vi "Panel Get Load Info.vi"(2 "file path (dialog if empty)":path) -> (6 "Load Type Out":string(combo), 8 "Nominal Load  Weight Out":string(combo))   [LabVIEW 2012]
uses:
  <vilib>/Utility/miscctls.llb/LVComboBoxStrsAndValuesArrayTypeDef.ctl
  <vilib>/Utility/file.llb/Read From Spreadsheet File (string).vi
panel:
  in  "error IO":errorcluster
  in  "Nominal Load  Weight (Select or Enter Value)":string(combo)
  in  "Load Type (Select or Enter Value)":string(combo)
  in  "stop":bool
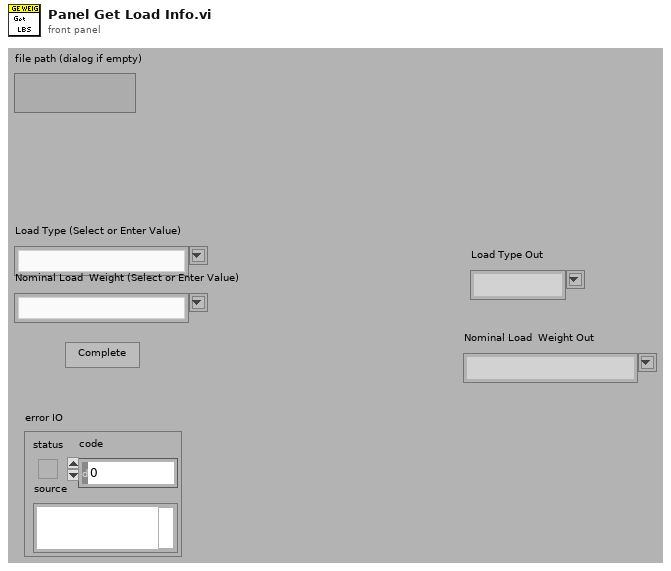
[diagram p1: front panel]
types:
  T1 = typedef "LVComboBoxStrsAndValuesArrayTypeDef.ctl" = cluster{"String":string, "Value":string}[]
  T2 = enum32{"Invalid", "Standard", "Closed", "Hidden", "Minimized", "Maximized"}
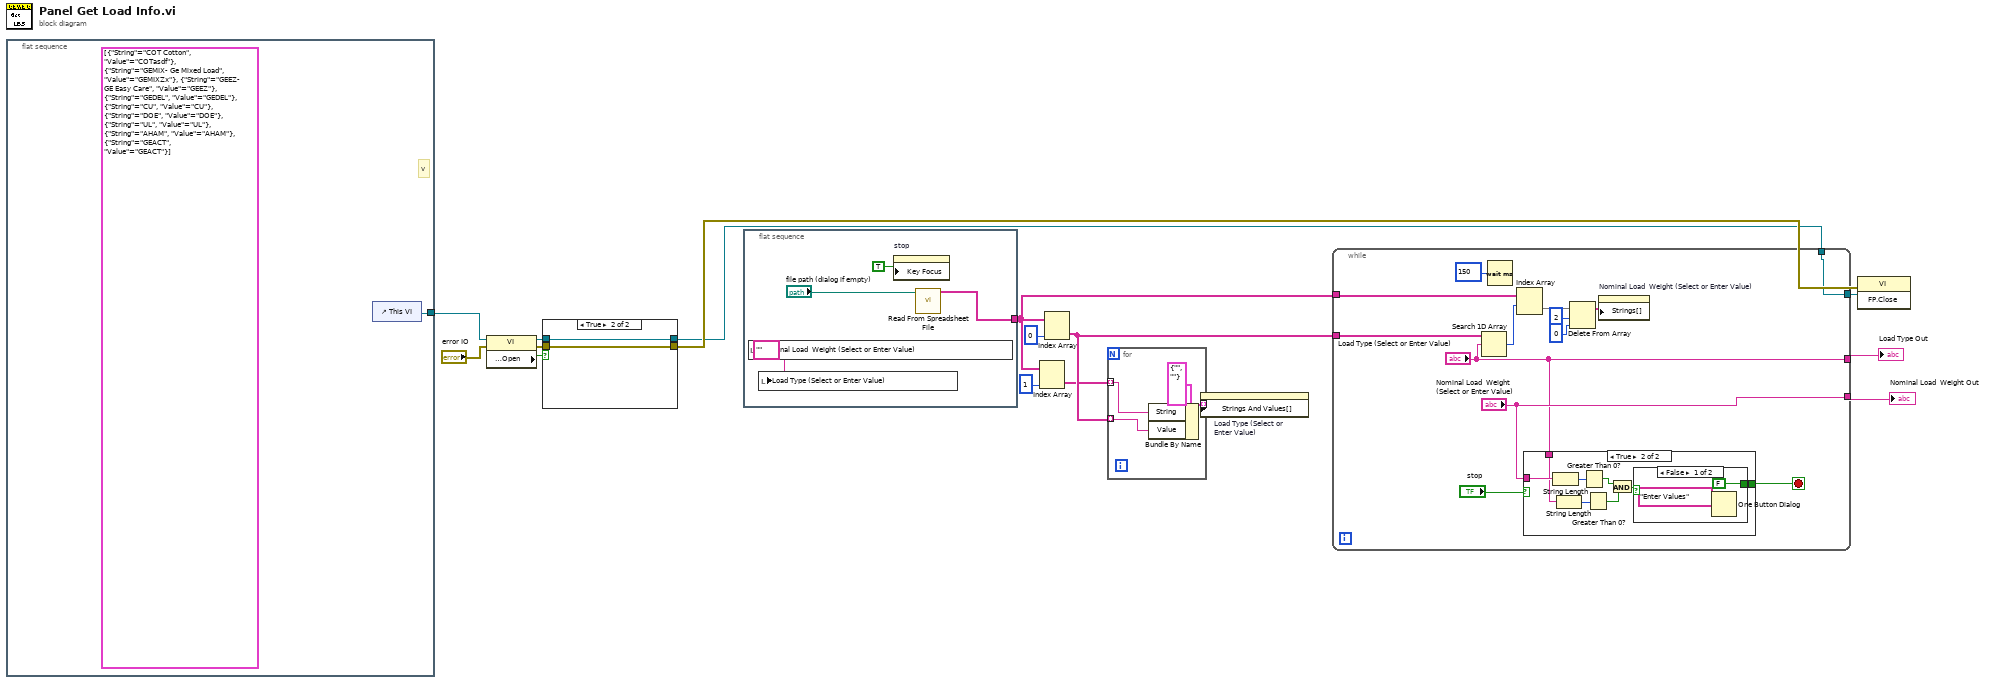
[diagram p0: block diagram]
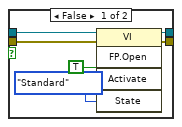
[diagram p2: hidden frame]
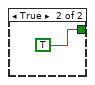
[diagram p4: hidden frame]
diagram:
  n1 = flat-sequence {
    tunnel: [w17] -> w6
    frame #0 {
      (unwired) T1 [{"String"="COT Cotton", "Value"="COTasdf"}, {"String"="GEMIX- Ge Mixed Load", "Value"="GEMIXZx"}, {"String"="GEEZ- GE Easy Care", "Value"="GEEZ"}, {"String"="GEDEL", "Value"="GEDEL"}, {"String"="CU", "Value"="CU"}, {"String"="DOE", "Value"="DOE"}, {"String"="UL", "Value"="UL"}, {"String"="AHAM", "Value"="AHAM"}, {"String"="GEACT", "Value"="GEACT"}] ("Strings And Values []")
      # "v"
      n2 = control-ref of="This VI"() -> (w17:refnum<vi>)
    }
  }
  n3 = property class="VI"(reference=w6, error in="error IO") -> (reference out=w8:refnum<vi>, error out=w9:errorcluster, "Front Panel.Open"=w7:bool)
  n4 = case shown="True" w7 {
    tunnel: [w21 w25] -> w12
    tunnel: w9 -> [w20 w25]
    tunnel: w8 -> [w19 w24]
    tunnel: [w18 w24] -> w10
    frame False {
      n5 = invoke class="VI" method="FP.Open"(reference=w19, error in=w20, "Activate"=TRUE, "State"=T2."Standard") -> (reference out=w18:refnum<vi>, error out=w21:errorcluster)  [unwired: 1 in, 3 out]
    }
    frame True {
    }
  }
  n6 = flat-sequence {
    tunnel: [w27] -> w3
    frame #0 {
      w29 = "" ("Load Type (Select or Enter Value)")
      n7 = local write "Nominal Load  Weight (Select or Enter Value)"(w29) -> ()
      n8 = local write "Load Type (Select or Enter Value)"(w29) -> ()
      n9 = property on="stop" class="Bool"("Key Focus"=TRUE) -> ()  [unwired: 2 in, 2 out]
      n10 = call-poly <vilib>:"Read From Spreadsheet File.vi"("file path (dialog if empty)"="file path (dialog if empty)") -> ("all rows"=w27:string[][])  [unwired: 6 in, 4 out]
    }
  }
  n11 = Index Array(array=w3, index (col)=1 ("disabled index (col)")) -> (element=w2:string[])  [unwired: 1 in]
  n12 = Index Array(array=w3, index (col)=0 ("disabled index (col)")) -> (element=w5:string[])  [unwired: 1 in]
  n13 = for {
    tunnel: w5 -> [w33] mode=indexing
    tunnel: w2 -> [w32] mode=indexing
    tunnel: [w30] -> w1 mode=indexing
    n14 = Bundle By Name(cluster=cluster{"String":string, "Value":string} {"String"="", "Value"=""} ("Cluster"), "String"=w32, "Value"=w33) -> (w30:cluster{"String":string, "Value":string})
  }
  n15 = property on="Load Type (Select or Enter Value)" class="CmbBox"("Strings And Values[]"=w1) -> ()  [unwired: 2 in, 2 out]
  n16 = while {
    tunnel: w5 -> [w45]
    tunnel: ["Load Type (Select or Enter Value)"] -> w15
    tunnel: w3 -> [w44]
    tunnel: ["Nominal Load  Weight (Select or Enter Value)"] -> w14
    tunnel: [w38] -> w11
    tunnel: w10 -> [w38]
    stop <- w34 stop-if-true
    n17 = Search 1D Array(1D array=w45, element="Load Type (Select or Enter Value)") -> (index of element=w43:i32)  [unwired: 1 in]
    n18 = Wait (ms)(milliseconds to wait=u32 150) -> ()  [unwired: 1 out]
    n19 = Index Array(array=w44, index (row)=w43) -> (element=w42:string[])  [unwired: 1 in]
    n20 = case shown="True" "stop" {
      selector: "stop" -> [w47 _]
      tunnel: "Nominal Load  Weight (Select or Enter Value)" -> [_ w51]
      tunnel: "Load Type (Select or Enter Value)" -> [_ w50]
      tunnel: [w47 w48] -> w34
      frame False {
      }
      frame True {
        n21 = String Length(string=w51) -> (length=w55:i32)
        n22 = String Length(string=w50) -> (length=w54:i32)
        n23 = Greater Than 0?(x=w55) -> (x > 0?=w53:bool)
        n24 = Greater Than 0?(x=w54) -> (x > 0?=w52:bool)
        n25 = And(x=w53, y=w52) -> (x .and. y?=w49:bool)
        n26 = case shown="False" w49 {
          tunnel: [FALSE TRUE] -> w48
          frame False {
            n27 = One Button Dialog(message="Enter Values") -> ()  [unwired: 1 in, 1 out]
          }
          frame True {
          }
        }
      }
    }
    n28 = Delete From Array(array=w42, length=2, index=0) -> (array with subset deleted=w39:string[])  [unwired: 1 out]
    n29 = property on="Nominal Load  Weight (Select or Enter Value)" class="CmbBox"("Strings[]"=w39) -> ()  [unwired: 2 in, 2 out]
  }
  "Load Type Out" <- w15
  "Nominal Load  Weight Out" <- w14
  n30 = invoke class="VI" method="FP.Close"(reference=w11, error in=w12) -> ()  [unwired: 1 in, 3 out]
